vi "静态字段(Write).vi"() -> ()   [LabVIEW 2013]
uses:
  Math.lvclass
panel:
  in  "停止":bool
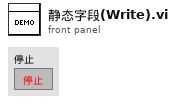
[diagram p1: front panel]
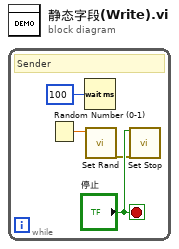
[diagram p0: block diagram]
diagram:
  n1 = while "While循环" {
    stop <- "停止" stop-if-true
    # "Sender"
    n2 = Random Number (0-1)() -> (number: 0 to 1=w2:dbl)
    n3 = Wait (ms)(milliseconds to wait=u32 100 ("等待时间（毫秒）")) -> ()  [unwired: 1 out]
    n4 = call "Set Rand.vi"("Rand"=w2) -> ("error out"=w1:errorcluster)  [unwired: 18 in]
    n5 = call "Set Stop.vi"("Stop"="停止", "error in (no error)"=w1) -> ()  [unwired: 17 in, 1 out]
  }
